vi "Agilent E3633A Init.vi"(6 "error in (no error)":errorcluster, 9 "resource name":refnum<k15>="GPIB0::5::INSTR") -> (0 "error out":errorcluster, 3 "instrument handle out":refnum<k15>="GPIB0::5::INSTR")   [LabVIEW 2016]
panel:
  out "CURR READ":string="+4.85360900E-04\n"
  in  "MEAS buffer":string="MEAS:CURR?"
  in  "Turn ON Output":string="OUTP ON"
  in  "write VOLT Buff":string="VOLT 20"
  out "Max Volt Limit":dbl=20.6 format="%.2p"
  in  "write CURR Buff":string="CURR 0"
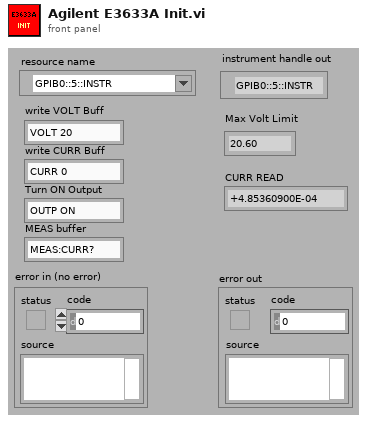
[diagram p1: front panel]
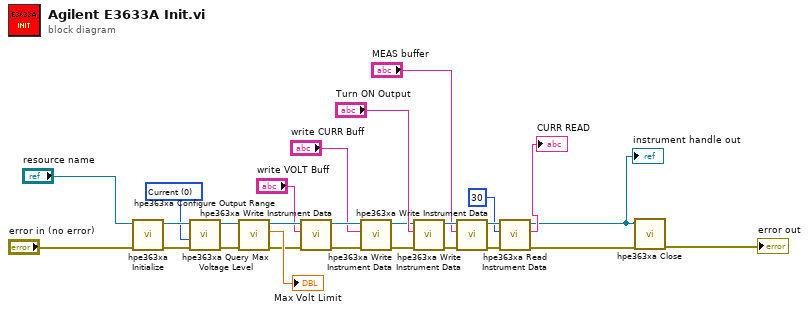
[diagram p0: block diagram]
diagram:
  w4 = 0 items=["Voltage"=1, "Current"=0] ("Range Type (Voltage)")
  n1 = call "hpe363xa Initialize.vi"("error in (no error)"="error in (no error)", "resource name"="resource name") -> ("error out"=w25:errorcluster, "instrument handle out"=w23:refnum<k15>)  [unwired: 8 in]
  n2 = call "hpe363xa Configure Output Range.vi"("error in (no error)"=w25, "Range Type (Voltage)"=w4, "instrument handle"=w23) -> ("error out"=w26:errorcluster, "instrument handle out"=w22:refnum<k15>)  [unwired: 7 in]
  n3 = call "hpe363xa Query Max Voltage Level.vi"("error in (no error)"=w26, "instrument handle"=w22) -> ("error out"=w18:errorcluster, "Max Voltage Level"=→"Max Volt Limit":dbl, "instrument handle out"=w20:refnum<k15>)  [unwired: 7 in]
  n4 = call "hpe363xa Write Instrument Data.vi"("error in (no error)"=w18, "Write Buffer"="write VOLT Buff", "instrument handle"=w20) -> ("error out"=w16:errorcluster, "instrument handle out"=w17:refnum<k15>)  [unwired: 7 in]
  n5 = call "hpe363xa Write Instrument Data.vi"("error in (no error)"=w16, "Write Buffer"="write CURR Buff", "instrument handle"=w17) -> ("error out"=w12:errorcluster, "instrument handle out"=w13:refnum<k15>)  [unwired: 7 in]
  n6 = call "hpe363xa Write Instrument Data.vi"("error in (no error)"=w12, "Write Buffer"="Turn ON Output", "instrument handle"=w13) -> ("error out"=w10:errorcluster, "instrument handle out"=w11:refnum<k15>)  [unwired: 7 in]
  n7 = call "hpe363xa Write Instrument Data.vi"("error in (no error)"=w10, "Write Buffer"="MEAS buffer", "instrument handle"=w11) -> ("error out"=w7:errorcluster, "instrument handle out"=w8:refnum<k15>)  [unwired: 7 in]
  n8 = call "hpe363xa Read Instrument Data.vi"("error in (no error)"=w7, "Number Of Bytes To Read (0)"=30 ("byte count"), "instrument handle"=w8) -> ("error out"=w3:errorcluster, "Read Buffer"=→"CURR READ":string, "instrument handle out"=w1:refnum<k15>)  [unwired: 5 in, 1 out]
  "instrument handle out" <- w1
  n9 = call "hpe363xa Close.vi"("error in (no error)"=w3, "instrument handle"=w1) -> ("error out"=→"error out":errorcluster)  [unwired: 9 in]
